vi "subObjectsToContent.vi"(7 "Expand containers?":bool, 11 "Items":refnum<class "ILabVIEWItem.lvclass">[](array[class])) -> (3 "Export string":string)   [LabVIEW 2020, in "DefaultExtensions.lvlib" / "CGrapherDGML.lvclass"]
uses:
  CGrapherDGML.lvclass
  obj/Addons/LabVIEWObjectInterfaces.lvlibp/LabVIEWObjectInterfaces/ILabVIEWItem/ILabVIEWItem.lvclass
  obj/Addons/LabVIEWObjectInterfaces.lvlibp/LabVIEWObjectInterfaces/IDependencyItemRule/IDependencyItemRule.lvclass
  dd3e3d63-517b-426a-9b3a-239d42afcb21.vi
  b950e2de-df04-4522-a07c-0797f8ba700f.vi
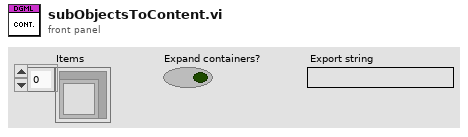
[diagram p1: front panel]
types:
  T1 = typedef "LabVIEWItem.lvlibp/CLabVIEWItem.lvclass/ConnectionSet.ctl" = set{string}
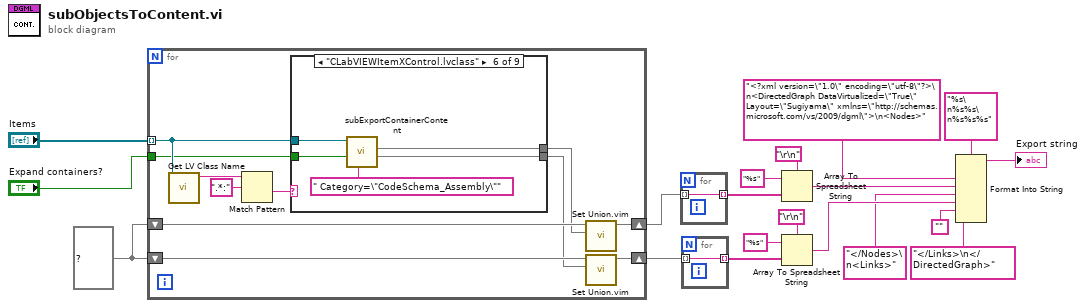
[diagram p0: block diagram]
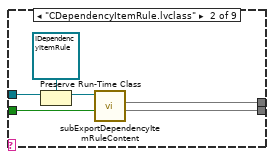
[diagram p3: hidden frame]
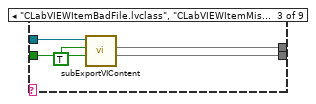
[diagram p4: hidden frame]
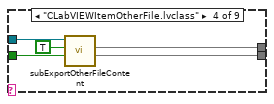
[diagram p5: hidden frame]
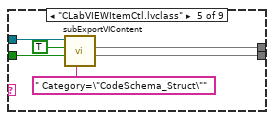
[diagram p6: hidden frame]
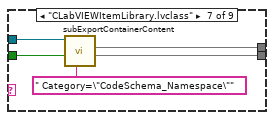
[diagram p7: hidden frame]
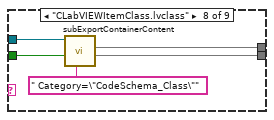
[diagram p8: hidden frame]
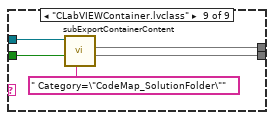
[diagram p9: hidden frame]
diagram:
  w16 = set{string} {} ("union")
  n1 = for {
    tunnel: "Items" -> [w30] mode=indexing
    shift-right: [w25] -> w18
    shift-left: w16 -> [w26]
    shift-right: [w23] -> w17
    shift-left: w16 -> [w24]
    tunnel: "Expand containers?" -> [w20]
    n2 = call <vilib>:"Get LV Class Name.vi"("object"=w30) -> ("class name"=w29:string)  [unwired: 9 in, 1 out]
    n3 = Match Pattern(string=w29, regular expression=".*:") -> (after substring=w27:string)  [unwired: 1 in, 3 out]
    n4 = case shown="\"CLabVIEWItemXControl.lvclass\"" w27 {
      tunnel: w30 -> [_ w36 w41 w46 w52 w57 w62 w67 w72]
      tunnel: [_ w33 w39 w44 w50 w56 w61 w66 w71] -> w22
      tunnel: [_ w32 w38 w43 w49 w55 w60 w65 w70] -> w21
      tunnel: w20 -> [_ w31 w37 w42 w47 w53 w58 w63 w68]
      frame Default {
      }
      frame "CDependencyItemRule.lvclass" {
        n5 = Preserve Run-Time Class(object in=w36, 2:refnum<class "IDependencyItemRule.lvclass"> refnum ("IDependencyItemRule in")) -> (object out=w34:refnum<class "IDependencyItemRule.lvclass">)  [unwired: 1 in, 1 out]
        n6 = call "subExportDependencyItemRuleContent.vi"("Expand?"=w31, "IDependencyItemRule in"=w34) -> ("Links"=w32:T1, "Nodes"=w33:T1)  [unwired: 6 in, 2 out]
      }
      frame "CLabVIEWItemBadFile.lvclass", "CLabVIEWItemMissingFile.lvclass", "CLabVIEWItemVI.lvclass", "CLabVIEWItemVIM.lvclass" {
        n7 = call "subExportVIContent.vi"("Expand?"=w37, "Add virtual folders?"=TRUE, "ILabVIEWItem in"=w41) -> ("Links"=w38:T1, "Nodes"=w39:T1)  [unwired: 5 in, 2 out]
      }
      frame "CLabVIEWItemOtherFile.lvclass" {
        n8 = call "subExportOtherFileContent.vi"("Expand?"=w42, "Add virtual folders?"=TRUE, "ILabVIEWItem in"=w46) -> ("Links"=w43:T1, "Nodes"=w44:T1)  [unwired: 5 in, 2 out]
      }
      frame "CLabVIEWItemCtl.lvclass" {
        n9 = call "subExportVIContent.vi"("CodeSchema"=" Category=\"CodeSchema_Struct\"", "Expand?"=w47, "Add virtual folders?"=TRUE, "ILabVIEWItem in"=w52) -> ("Links"=w49:T1, "Nodes"=w50:T1)  [unwired: 4 in, 2 out]
      }
      frame "CLabVIEWItemXControl.lvclass" {
        n10 = call "subExportContainerContent.vi"("CodeSchema"=" Category=\"CodeSchema_Assembly\"", "Expand?"=w53, "ILabVIEWItem in"=w57) -> ("Links"=w55:T1, "Nodes"=w56:T1)  [unwired: 5 in, 2 out]
      }
      frame "CLabVIEWItemLibrary.lvclass" {
        n11 = call "subExportContainerContent.vi"("CodeSchema"=" Category=\"CodeSchema_Namespace\"", "Expand?"=w58, "ILabVIEWItem in"=w62) -> ("Links"=w60:T1, "Nodes"=w61:T1)  [unwired: 5 in, 2 out]
      }
      frame "CLabVIEWItemClass.lvclass" {
        n12 = call "subExportContainerContent.vi"("CodeSchema"=" Category=\"CodeSchema_Class\"", "Expand?"=w63, "ILabVIEWItem in"=w67) -> ("Links"=w65:T1, "Nodes"=w66:T1)  [unwired: 5 in, 2 out]
      }
      frame "CLabVIEWContainer.lvclass" {
        n13 = call "subExportContainerContent.vi"("CodeSchema"=" Category=\"CodeMap_SolutionFolder\"", "Expand?"=w68, "ILabVIEWItem in"=w72) -> ("Links"=w70:T1, "Nodes"=w71:T1)  [unwired: 5 in, 2 out]
      }
    }
    n14 = call "Set Union.vim"("set 2"=w22, "set 1"=w26) -> ("union"=w25:set{string})  [unwired: 9 in]
    n15 = call "Set Union.vim"("set 2"=w21, "set 1"=w24) -> ("union"=w23:set{string})  [unwired: 9 in]
  }
  n16 = for {
    tunnel: [w73] -> w12 mode=indexing
    tunnel: w18 -> [w73] mode=indexing
  }
  n17 = for {
    tunnel: [w74] -> w13 mode=indexing
    tunnel: w17 -> [w74] mode=indexing
  }
  n18 = Array To Spreadsheet String(delimiter (Tab)="\r\n", array=w12, 3:"%s" ("format string")) -> (spreadsheet string=w7:string)
  n19 = Array To Spreadsheet String(delimiter (Tab)="\r\n", array=w13, 3:"%s" ("format string")) -> (spreadsheet string=w10:string)
  n20 = Format Into String(format string="%s\n%s%s\n%s%s%s", "<?xml version=\"1.0\" encoding=\"utf-8\"?>\n<DirectedGraph DataVirtualized=\"True\" Layout=\"Sugiyama\" xmlns=\"http://schemas.microsoft.com/vs/2009/dgml\">\n<Nodes>", w7, "</Nodes>\n<Links>" ("format string"), w10, "", "</Links>\n</DirectedGraph>") -> (resulting string=→"Export string":string)  [unwired: 2 in, 1 out]
